vi "QUDI_QPD_PID_basic.vi"() -> ()   [LabVIEW 2015]
uses:
  <vilib>/rvi/Analysis/control/PID/Typedef/niFpgaPID_PIGains.ctl
  <vilib>/Platform/TimedLoop/XDataNode/timing_clust.ctl
  <vilib>/Platform/TimedLoop/XDataNode/nitl_modes.ctl
  <vilib>/Platform/TimedLoop/XDataNode/wakeup.ctl
  <vilib>/rvi/FXPMathLib/basic elements/FxpIntAccumulator/subVIs/nifxpmath_IntAccumulator_SimConfig.ctl
  <vilib>/rvi/Emulation/niFpgaGetClockAttributes.vi
  <vilib>/rvi/Emulation/niFpgaSctlEmulationGetInTimedLoop.vi
  <vilib>/rvi/Emulation/niFpgaEmulationReportErrorSimple.vi
  <vilib>/rvi/eio/common/nirviEmuTemplateMethod_errors.vi
  <vilib>/rvi/Emulation/niFpgaProcessEmulError.vi
  <vilib>/rvi/Analysis/common/codeGenErrors/XNode/niFpgaXNodeCodeGenErrorHandle.vi
  <vilib>/rvi/Emulation/niFpgaCriticalErrorInLSC.vi
  <vilib>/rvi/FXPMathLib/basic elements/FxpIntAccumulator/simVIs/DllFxpIntAccumulator_sub.vi
  <vilib>/rvi/Analysis/control/PID/SubVIs/niFpgaPID_PIWrapper.vi
  <vilib>/eio/EIONode/EIONode.xnode
  <vilib>/rvi/Analysis/measure/dc-rms/XNode/niFpgaDC-RMS.xnode
  <vilib>/Platform/TimedLoop/XDataNode/XDataNode.xnode
  <vilib>/rvi/FXPMathLib/basic elements/FxpIntAccumulator/XNode/nifxpmath_IntAccumulator.xnode
  <vilib>/Platform/TimedLoop/XDataNode/XDNodeRunTimeDep.lvlib
panel:
  in  "ref_axis":bool
  out "output":i16
  in  "I":i16
  in  "P":i16
  in  "reset":bool
  in  "setpoint":i16
  in  "autofocus":bool
  out "counter":u32
  out "Sum":i16
  out "Y":i16
  out "X":i16
  in  "integration_time_us":u16=100 caption="Count(uSec)"
  in  "stop":bool
  out "duration_ms":u16
  in  "reset_counter":bool
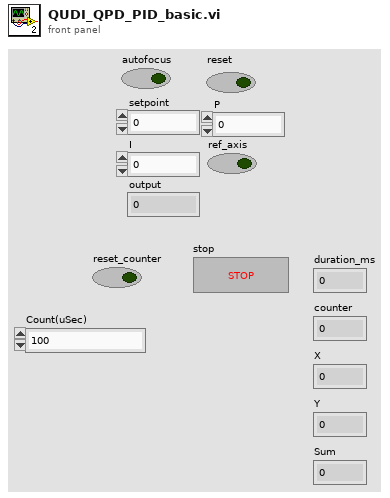
[diagram p1: front panel]
types:
  T1 = typedef "niFpgaPID_PIGains.ctl" = cluster{"proportional gain":sgl, "integral gain":sgl}
  T2 = typedef "XDNodeRunTimeDep.lvlib/timing_clust.ctl" = cluster{"Expected End [f-1]":u64, "Actual End [f-1]":u64, "Finished Late? [f-1]":bool, "Expected End [i-1]":u64, "Actual End [i-1]":u64, "Finished Late? [i-1]":bool, "Expected Start [i]":u64, "Actual Start [i]":u64, "Expected Start [f]":u64, "Actual Start [f]":u64, "Source Name":string, "Structure Name":string, "Period":i64, "Deadline":i64, "Offset":i64, "Start":i64, "Priority":i32, "Timeout":i32, "Mode":T3, "Wakeup Reason":T4, "Error":errorcluster, "Source Type":string, "Secondary Source Type":string, "Global End Time":u64, "Global Start Time":u64, "Frame Duration":u64, "Iteration Duration":u64, "Assigned CPU":i32, "I/O Scan Engine Mode":u32}
  T3 = typedef "XDNodeRunTimeDep.lvlib/nitl_modes.ctl" = enum32{"No Change", "Process missed periods, maintain original phase", "Discard missed periods, maintain original phase", "Process missed periods, ignore original phase", "Discard missed periods, ignore original phase"}
  T4 = typedef "XDNodeRunTimeDep.lvlib/wakeup.ctl" = enum32{"Normal", "Aborted", "Asynchronous wakeup", "Timing source error", "Timed loop error", "Timeout"}
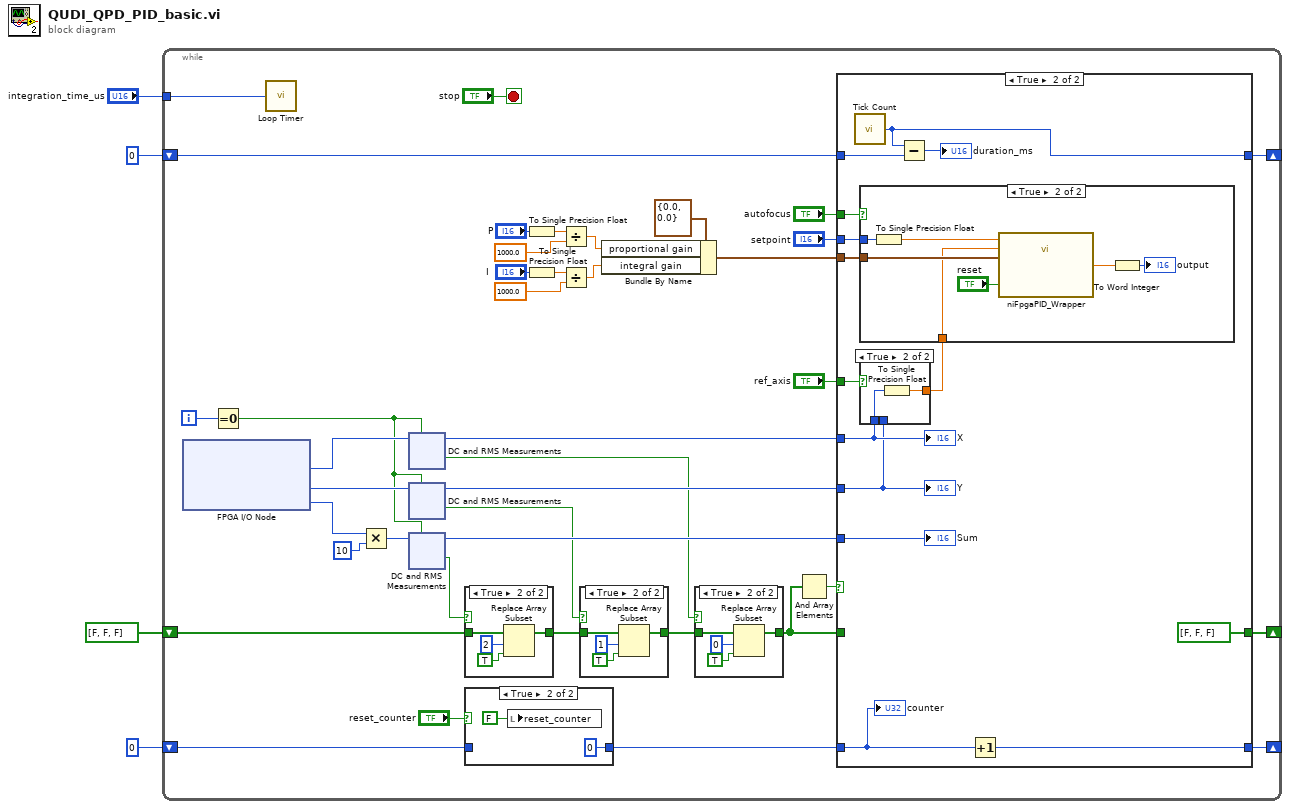
[diagram p0: block diagram]
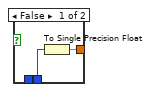
[diagram p7: hidden frame]
diagram:
  n1 = while {
    shift-right: [w28] -> _
    shift-left: bool[] [FALSE, FALSE, FALSE] ("initialized array") -> [w36]
    shift-right: [w26] -> _
    shift-left: u16 0 -> [w27]
    tunnel: "integration_time_us" -> [w25]
    shift-right: [w24] -> _
    shift-left: u32 0 -> [w22]
    i -> [w42]
    stop <- "stop" stop-if-true
    n2 = xnode "FPGA I/O Node"() -> ("Connector0/AI0"=w44:i16, "Connector0/AI1"=w40:i16, "Connector0/AI2"=w7:i16)  [unwired: 3 in, 3 out]
    n3 = Equal To 0?(x=w42) -> (x = 0?=w37:bool)
    n4 = call "Loop Timer"("Count(uSec)"=w25) -> ()  [unwired: 1 out]
    n5 = Multiply(x=w7, y=i16 10) -> (x*y=w6:i16)
    n6 = xnode "DC and RMS Measurements"("input data"=w44, "reset"=w37) -> ("DC"=w41:i16, "output valid"=w31:bool)
    n7 = xnode "DC and RMS Measurements"("input data"=w40, "reset"=w37) -> ("DC"=w39:i16, "output valid"=w32:bool)
    n8 = xnode "DC and RMS Measurements"("input data"=w6, "reset"=w37) -> ("DC"=w38:i16, "output valid"=w33:bool)
    n9 = case shown="True" w33 {
      tunnel: w36 -> [w53 w56]
      tunnel: [w53 w54] -> w35
      frame False {
      }
      frame True {
        n10 = Replace Array Subset(array=w56, new element=TRUE, index=2) -> (w54:bool[])
      }
    }
    n11 = case shown="True" "reset_counter" {
      tunnel: w22 -> [w45 _]
      tunnel: [w45 u32 0] -> w21
      frame False {
      }
      frame True {
        n12 = local write "reset_counter"(FALSE ("Reset counter")) -> ()
      }
    }
    n13 = To Single Precision Float(number="P") -> (single precision float=w14:sgl)
    n14 = To Single Precision Float(number="I") -> (single precision float=w11:sgl)
    n15 = Divide(x=w14, y=sgl 1000.0) -> (x/y=w12:sgl)
    n16 = Divide(x=w11, y=sgl 1000.0) -> (x/y=w9:sgl)
    n17 = case shown="True" w32 {
      tunnel: w35 -> [w58 w61]
      tunnel: [w58 w59] -> w34
      frame False {
      }
      frame True {
        n18 = Replace Array Subset(array=w61, new element=TRUE, index=1) -> (w59:bool[])
      }
    }
    n19 = Bundle By Name(cluster=T1 {"proportional gain"=0.0, "integral gain"=0.0} ("gains"), "proportional gain"=w12, "integral gain"=w9) -> (w15:T1)
    n20 = case shown="True" w31 {
      tunnel: [w48 w50] -> w29
      tunnel: w34 -> [w48 w49]
      frame False {
      }
      frame True {
        n21 = Replace Array Subset(array=w49, new element=TRUE, index=0) -> (w50:bool[])
      }
    }
    n22 = And Array Elements(Boolean array=w29) -> (logical AND=w30:bool)
    n23 = case shown="True" w30 {
      tunnel: w41 -> [_ w68]
      tunnel: w39 -> [_ w66]
      tunnel: w38 -> [_ w74]
      tunnel: w29 -> [w65 _]
      tunnel: [w65 bool[] [FALSE, FALSE, FALSE] ("initialized array")] -> w28
      tunnel: w27 -> [w64 w78]
      tunnel: [w64 w76] -> w26
      tunnel: w21 -> [w63 w73]
      tunnel: [w63 w75] -> w24
      tunnel: "autofocus" -> [_ w72]
      tunnel: "setpoint" -> [_ w71]
      tunnel: w15 -> [_ w70]
      tunnel: "ref_axis" -> [_ w69]
      frame False {
      }
      frame True {
        n24 = call "Tick Count"() -> ("Tick Count(mSec)"=w76:u16)
        n25 = case shown="True" w69 {
          tunnel: w68 -> [_ w83]
          tunnel: [w80 w82] -> w67
          tunnel: w66 -> [w81 _]
          frame False {
            n26 = To Single Precision Float(number=w81) -> (single precision float=w80:sgl)
          }
          frame True {
            n27 = To Single Precision Float(number=w83) -> (single precision float=w82:sgl)
          }
        }
        n28 = case shown="True" w72 {
          tunnel: w71 -> [_ w90]
          tunnel: w70 -> [_ w88]
          tunnel: w67 -> [_ w84]
          frame False {
          }
          frame True {
            n29 = To Single Precision Float(number=w90) -> (single precision float=w89:sgl)
            n30 = call-poly <vilib>:"niFpgaPID_Wrapper.vi"("setpoint"=w89, "reset? (F)"="reset", "process variable"=w84, "gains"=w88) -> ("output"=w86:sgl)  [unwired: 9 in, 2 out]
            n31 = To Word Integer(number=w86) -> (16bit integer=→"output":i16)
          }
        }
        n32 = Subtract(x=w76, y=w78) -> (x-y=→"duration_ms":u16)
        n33 = Increment(x=w73) -> (x+1=w75:u32)
        "X" <- w68
        "Y" <- w66
        "Sum" <- w74
        "counter" <- w73
      }
    }
  }
